vi "Check if Package is Upgradable Force Locked.vi"(8 "error in":errorcluster, 11 "package name":string) -> (0 "error out":errorcluster, 1 "upgradable?":bool, 2 "version to upgrade to":string, 3 "package name out":string, 4 "currently installed version":string)   [LabVIEW 2022 SP3, in "NIPM_Functions.lvlib"]
doc: "Checks whether an installed package has an upgrade available in any registered feeds\n\nINPUT(s)\n<B>Package name</B>: Specifies the package name\n\nOUTPUT(s)\n<B>Package name out</B>: Outputs the package name\n\n<B>Version to upgrade to</B>: Outputs the latest version to which you can upgrade the specified package\n\n<B>Upgradable?</B>: Outputs whether the specified package has an upgrade available in any registered feeds\n\n<B>Currently installed version</B>: Outputs the currently installed version (if any) of the specified package\n\nNIPM API 3.2.1.9\nNational Instruments\nCopyright (c) 2020, National Instruments"
uses:
  NIPM_Functions.lvlib
  <vilib>/National Instruments/NIPM API (Beta)/NIPM_API.lvlib
panel:
  out "cmd standard output":string
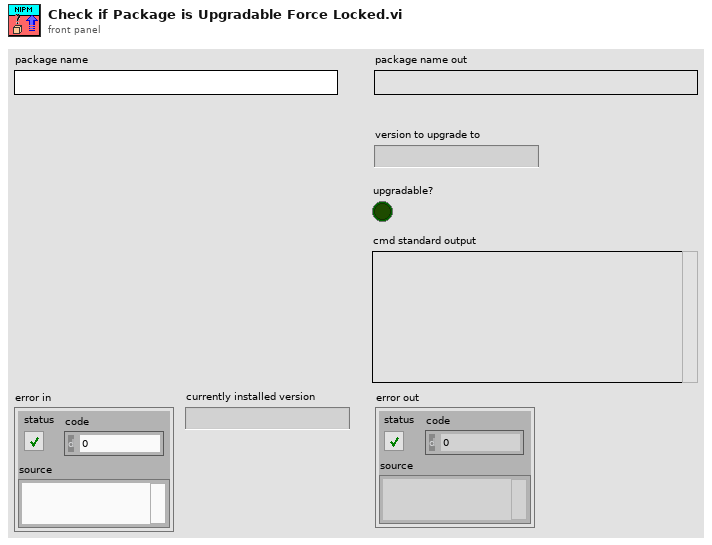
[diagram p1: front panel]
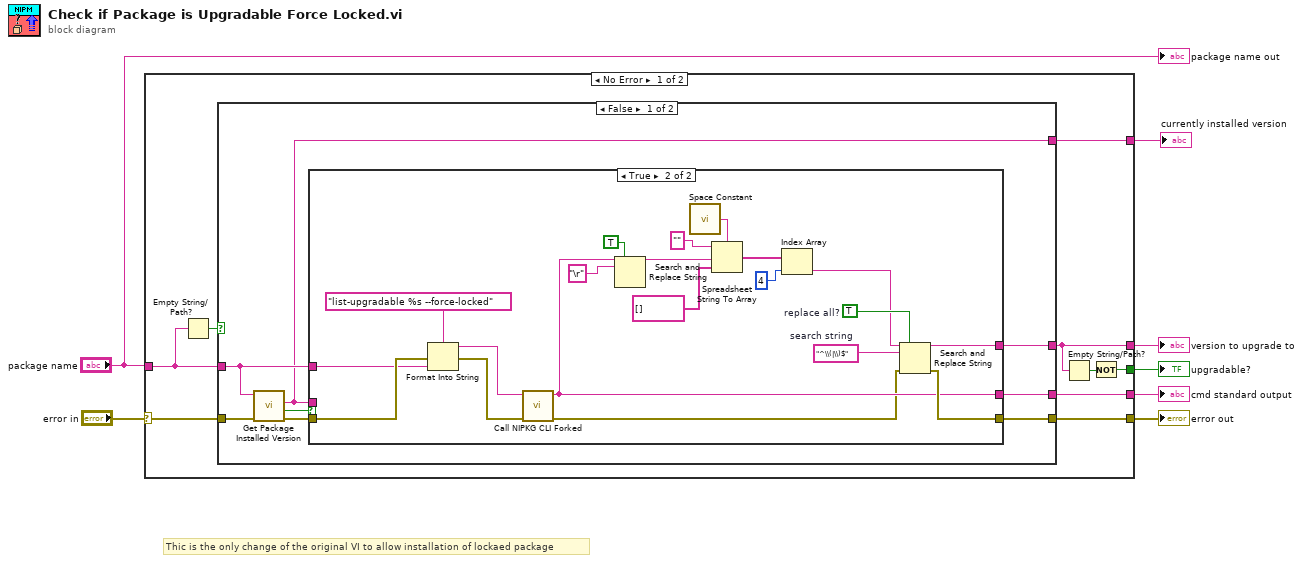
[diagram p0: block diagram]
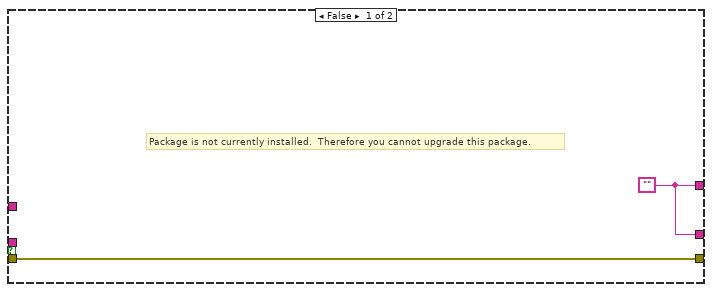
[diagram p2: hidden frame]
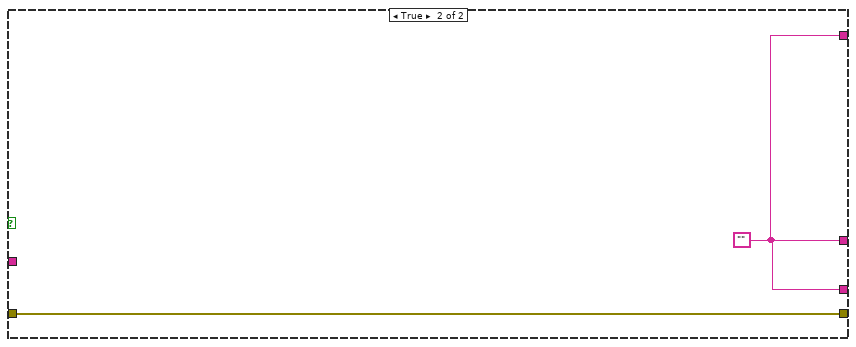
[diagram p3: hidden frame]
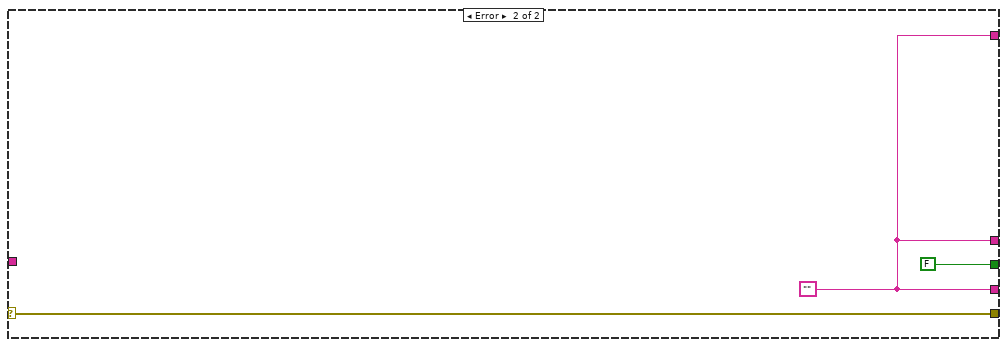
[diagram p4: hidden frame]
diagram:
  # "Thic is the only change of the original VI to allow installation of lockaed package"
  n1 = case shown="No Error" "error in" {
    selector: "error in" -> [w16 w51]
    tunnel: [w15 w49] -> w6
    tunnel: [w14 w51] -> w5
    tunnel: "package name" -> [w13 _]
    tunnel: [w11 w49] -> w3
    tunnel: [w9 FALSE] -> w2
    tunnel: [w8 w49] -> w1
    frame No Error {
      n2 = Empty String/Path?(string/path=w13) -> (empty?=w12:bool)
      n3 = case shown="False" w12 {
        tunnel: w16 -> [w21 w48]
        tunnel: [w23 w47] -> w15
        tunnel: [w22 w47] -> w11
        tunnel: [w24 w48] -> w14
        tunnel: w13 -> [w19 _]
        tunnel: [w17 w47] -> w8
        frame False {
          n4 = call <vilib>:"Get Package Installed Version.vi"("error in"=w21, "package name"=w19) -> ("error out"=w20:errorcluster, "installed?"=w18:bool, "installed version"=w17:string)  [unwired: 6 in, 1 out]
          n5 = case shown="True" w18 {
            tunnel: [w26 w31] -> w24
            tunnel: [w25 w29] -> w23
            tunnel: [w25 w32] -> w22
            tunnel: w20 -> [w26 w35]
            tunnel: w19 -> [_ w34]
            tunnel: w17 -> [_ _]
            frame False {
              w25 = "" ("standard output")
              # "Package is not currently installed.  Therefore you cannot upgrade this package."
            }
            frame True {
              w38 = TRUE  # replace all?
              w37 = "^\\(|\\)$"  # search string
              n6 = Format Into String(format string="list-upgradable %s --force-locked", error in=w35, w34) -> (resulting string=w30:string, error out=w27:errorcluster)  [unwired: 1 in]
              n7 = call "Call NIPKG CLI Forked.vi"("error in (no error)"=w27, "command"=w30) -> ("error out"=w28:errorcluster, "command line standard output"=w29:string)  [unwired: 8 in]
              n8 = Search and Replace String(replace all?=TRUE ("replace all? (F)"), input string=w29, search string="\r") -> (result string=w41:string)  [unwired: 5 in, 3 out]
              n9 = call <vilib>:"Space Constant.vi"() -> ("String"=w44:string)
              n10 = Spreadsheet String To Array(delimiter (Tab)=w44, format string="", spreadsheet string=w41, array type (2D Dbl)=string[] []) -> (array=w39:string[])
              n11 = Index Array(array=w39, index=4) -> (element=w36:string)
              n12 = Search and Replace String(replace all?=w38, input string=w36, search string=w37, error in=w28) -> (result string=w32:string, error out=w31:errorcluster)  [unwired: 4 in, 2 out]
            }
          }
        }
        frame True {
          w47 = ""
        }
      }
      n13 = Empty String/Path?(string/path=w11) -> (empty?=w10:bool)
      n14 = Not(x=w10) -> (.not. x?=w9:bool)
    }
    frame Error {
      w49 = "" ("standard output")
    }
  }
  "error out" <- w5
  "cmd standard output" <- w6
  "version to upgrade to" <- w3
  "upgradable?" <- w2
  "currently installed version" <- w1
  "package name out" <- "package name"
